vi "Compile Driver Configuration.vi"(8 "error in (no error)":errorcluster, 11 "Device Ref in":T1 format="%.0x") -> (0 "error out":errorcluster, 2 "Driver Configuration":T2, 3 "Device Ref out":T1 format="%.0x")   [LabVIEW 2017, in "NI-SWITCH System Explorer.lvlib"]
uses:
  NI-SWITCH System Explorer.lvlib
  Shared/Driver Configuration.ctl
  <vilib>/NI Veristand/Custom Device API/Custom Device Item Ref.ctl
  Scripting/SLSC Switch Scripting.lvlib
  Shared/NI-SWITCH Shared.lvlib
  <vilib>/NI VeriStand/Custom Device API/Custom Device API.lvlib
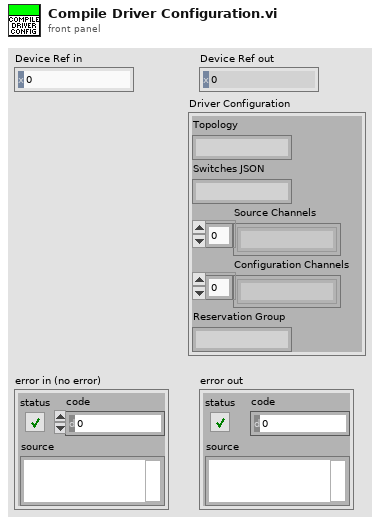
[diagram p1: front panel]
types:
  T1 = typedef "Custom Device API.lvlib/Custom Device Item Ref.ctl" = u64
  T2 = typedef "NI-SWITCH Shared.lvlib/Driver Configuration.ctl" = cluster{"Topology":string, "Switches JSON":string, "Source Channels":string[], "Configuration Channels":string[], "Reservation Group":string}
  T3 = typedef "SLSC Switch Scripting.lvlib/SLSC Switch All Properties.ctl" = cluster{"Product Name":string, "Topology":string, "Switches JSON":string, "Description":string, "Reservation Group":string}
  T4 = typedef "NI-SWITCH Shared.lvlib/Endpoint Configuration Cluster.ctl" = cluster{"Endpoint":string, "Configuration":T5}
  T5 = typedef "NI-SWITCH Shared.lvlib/Endpoint Configuration Enum.ctl" = enum16{"Load", "Source", "Configuration"}
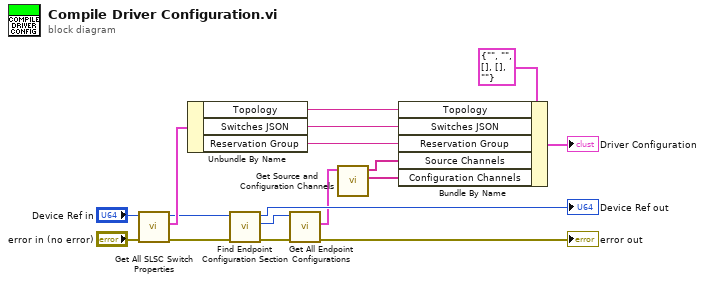
[diagram p0: block diagram]
diagram:
  n1 = call "Get All SLSC Switch Properties.vi"("error in"="error in (no error)", "slsc switch custom device in"="Device Ref in") -> ("error out"=w2:errorcluster, "properties"=w12:T3, "slsc switch custom device out"=w3:T1)  [unwired: 7 in]
  n2 = Unbundle By Name(w12) -> ("Topology"=w14:string, "Switches JSON"=w15:string, "Reservation Group"=w1:string)
  n3 = call "Find Endpoint Configuration Section.vi"("error in"=w2, "slsc switch custom device in"=w3) -> ("error out"=w9:errorcluster, "endpoint configuration"=w8:T1, "slsc switch custom device out"=→"Device Ref out":T1)  [unwired: 7 in]
  n4 = call "Get All Endpoint Configurations.vi"("error in"=w9, "endpoint configuration in"=w8) -> ("error out"=→"error out":errorcluster, "endpoint configurations"=w6:T4[])  [unwired: 7 in, 1 out]
  n5 = call "Get Source and Configuration Channels.vi"("All Endpoint Configurations"=w6) -> ("Configuration Channels"=w4:string[], "Source Channels"=w5:string[])  [unwired: 9 in]
  n6 = Bundle By Name(cluster=T2 {"Topology"="", "Switches JSON"="", "Source Channels"=[], "Configuration Channels"=[], "Reservation Group"=""} ("Driver Configuration"), "Topology"=w14, "Switches JSON"=w15, "Reservation Group"=w1, "Source Channels"=w5, "Configuration Channels"=w4) -> (→"Driver Configuration":T2)
